vi "PXI_Host_LargeFXP_Write_OldMethod_Benchmark.vi"() -> ()   [LabVIEW 2018]
uses:
  <vilib>/Platform/TimedLoop/XDataNode/timing_clust.ctl
  <vilib>/Platform/TimedLoop/XDataNode/nitl_modes.ctl
  <vilib>/Platform/TimedLoop/XDataNode/wakeup.ctl
  <vilib>/NI/LVFPGA Adv Session Resources/OpenByNameSubVI.vi
  <vilib>/rvi/interface/common/dynamic/niFpgaEscapeDelimiterAndNull.vi
  <vilib>/Utility/error.llb/Error Cluster From Error Code.vi
  <vilib>/rvi/errors/niLvFpgaAdjustHostInterfaceError.vi
  <vilib>/FPGAPlugInAG/Dynamic/niLvFpga_Close_Dynamic.vi
  <vilib>/platform/TimedLoop/XDataNode/XDataNode.xnode
  <vilib>/NI/LVFPGA Adv Session Resources/OpenByName.xnode
  <vilib>/rvi/interface/nirviReadWriteControl/nirviReadWriteControl.xnode
  <vilib>/rvi/interface/nirviCloseFPGA/nirviCloseFPGA.xnode
  NiFpgaLv.dll
  <vilib>/rvi/interface/Simulation/niFpgaSimulationCallBeginRW.vi
  <vilib>/NI/LVFPGA Adv Session Resources/LVFPGAAdvSessionResources.lvlib
  cRIO RT/FPGA Bitfile Register Operations/Scalar IO Operations/FPGA Register IO.lvlib
  <vilib>/Platform/TimedLoop/XDataNode/XDNodeRunTimeDep.lvlib
panel:
  out "Maximum(s)":dbl
  out "Standard deviation":dbl
  out "Waveform Graph":dbl[](graph)
  out "error out":errorcluster
  out "Execution time (s)":dbl
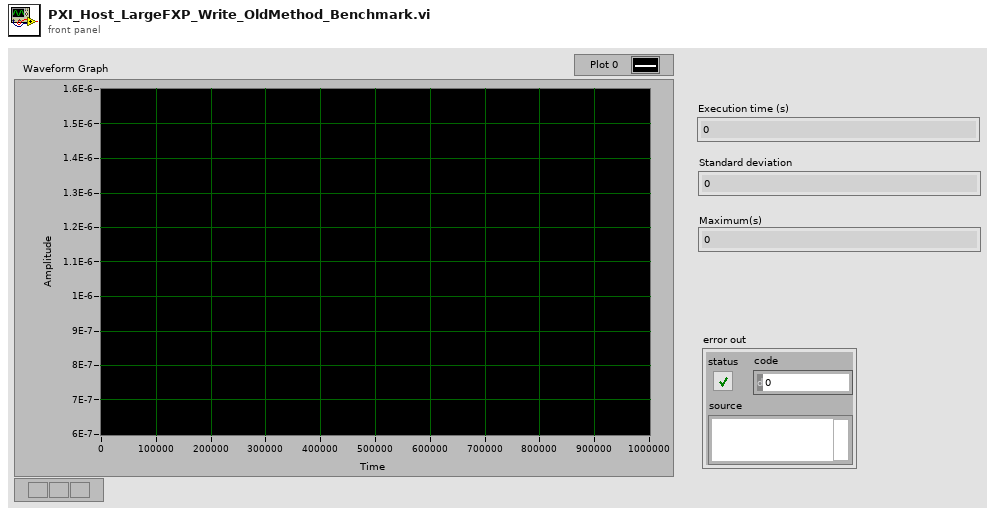
[diagram p1: front panel]
types:
  T1 = typedef "XDNodeRunTimeDep.lvlib/timing_clust.ctl" = cluster{"Expected End [f-1]":u64, "Actual End [f-1]":u64, "Finished Late? [f-1]":bool, "Expected End [i-1]":u64, "Actual End [i-1]":u64, "Finished Late? [i-1]":bool, "Expected Start [i]":u64, "Actual Start [i]":u64, "Expected Start [f]":u64, "Actual Start [f]":u64, "Source Name":string, "Structure Name":string, "Period":i64, "Deadline":i64, "Offset":i64, "Start":i64, "Priority":i32, "Timeout":i32, "Mode":T2, "Wakeup Reason":T3, "Error":errorcluster, "Source Type":string, "Secondary Source Type":string, "Global End Time":u64, "Global Start Time":u64, "Frame Duration":u64, "Iteration Duration":u64, "Assigned CPU":i32, "I/O Scan Engine Mode":u32}
  T2 = typedef "XDNodeRunTimeDep.lvlib/nitl_modes.ctl" = enum32{"No Change", "Process missed periods, maintain original phase", "Discard missed periods, maintain original phase", "Process missed periods, ignore original phase", "Discard missed periods, ignore original phase"}
  T3 = typedef "XDNodeRunTimeDep.lvlib/wakeup.ctl" = enum32{"Normal", "Aborted", "Asynchronous wakeup", "Timing source error", "Timed loop error", "Timeout"}
  T4 = cluster{"Name":string, "Depth":u32, "Write? (Deprecated:Use Implementation)":bool, "Physical Channel":u32, "Base Address":u32, "Data Width":u32, "Data Type":enum32{"Boolean", "I8", "I16", "I32", "I64", "U8", "U16", "U32", "U64", "FXP", "CustomControl", "SGL"}, "FXP Properties":variant, "Write Window Address":u32, "Implementation":enum16{"niFpgaTargetToHost", "niFpgaHostToTarget", "niFpgaPeerToPeerWriter", "niFpgaPeerToPeerReader", "niCoreTargetToHost", "niCoreHostToTarget"}, "Control Set":u32}[]
  T5 = cluster{"Name":string, "type":variant, "indicator?":bool}[]
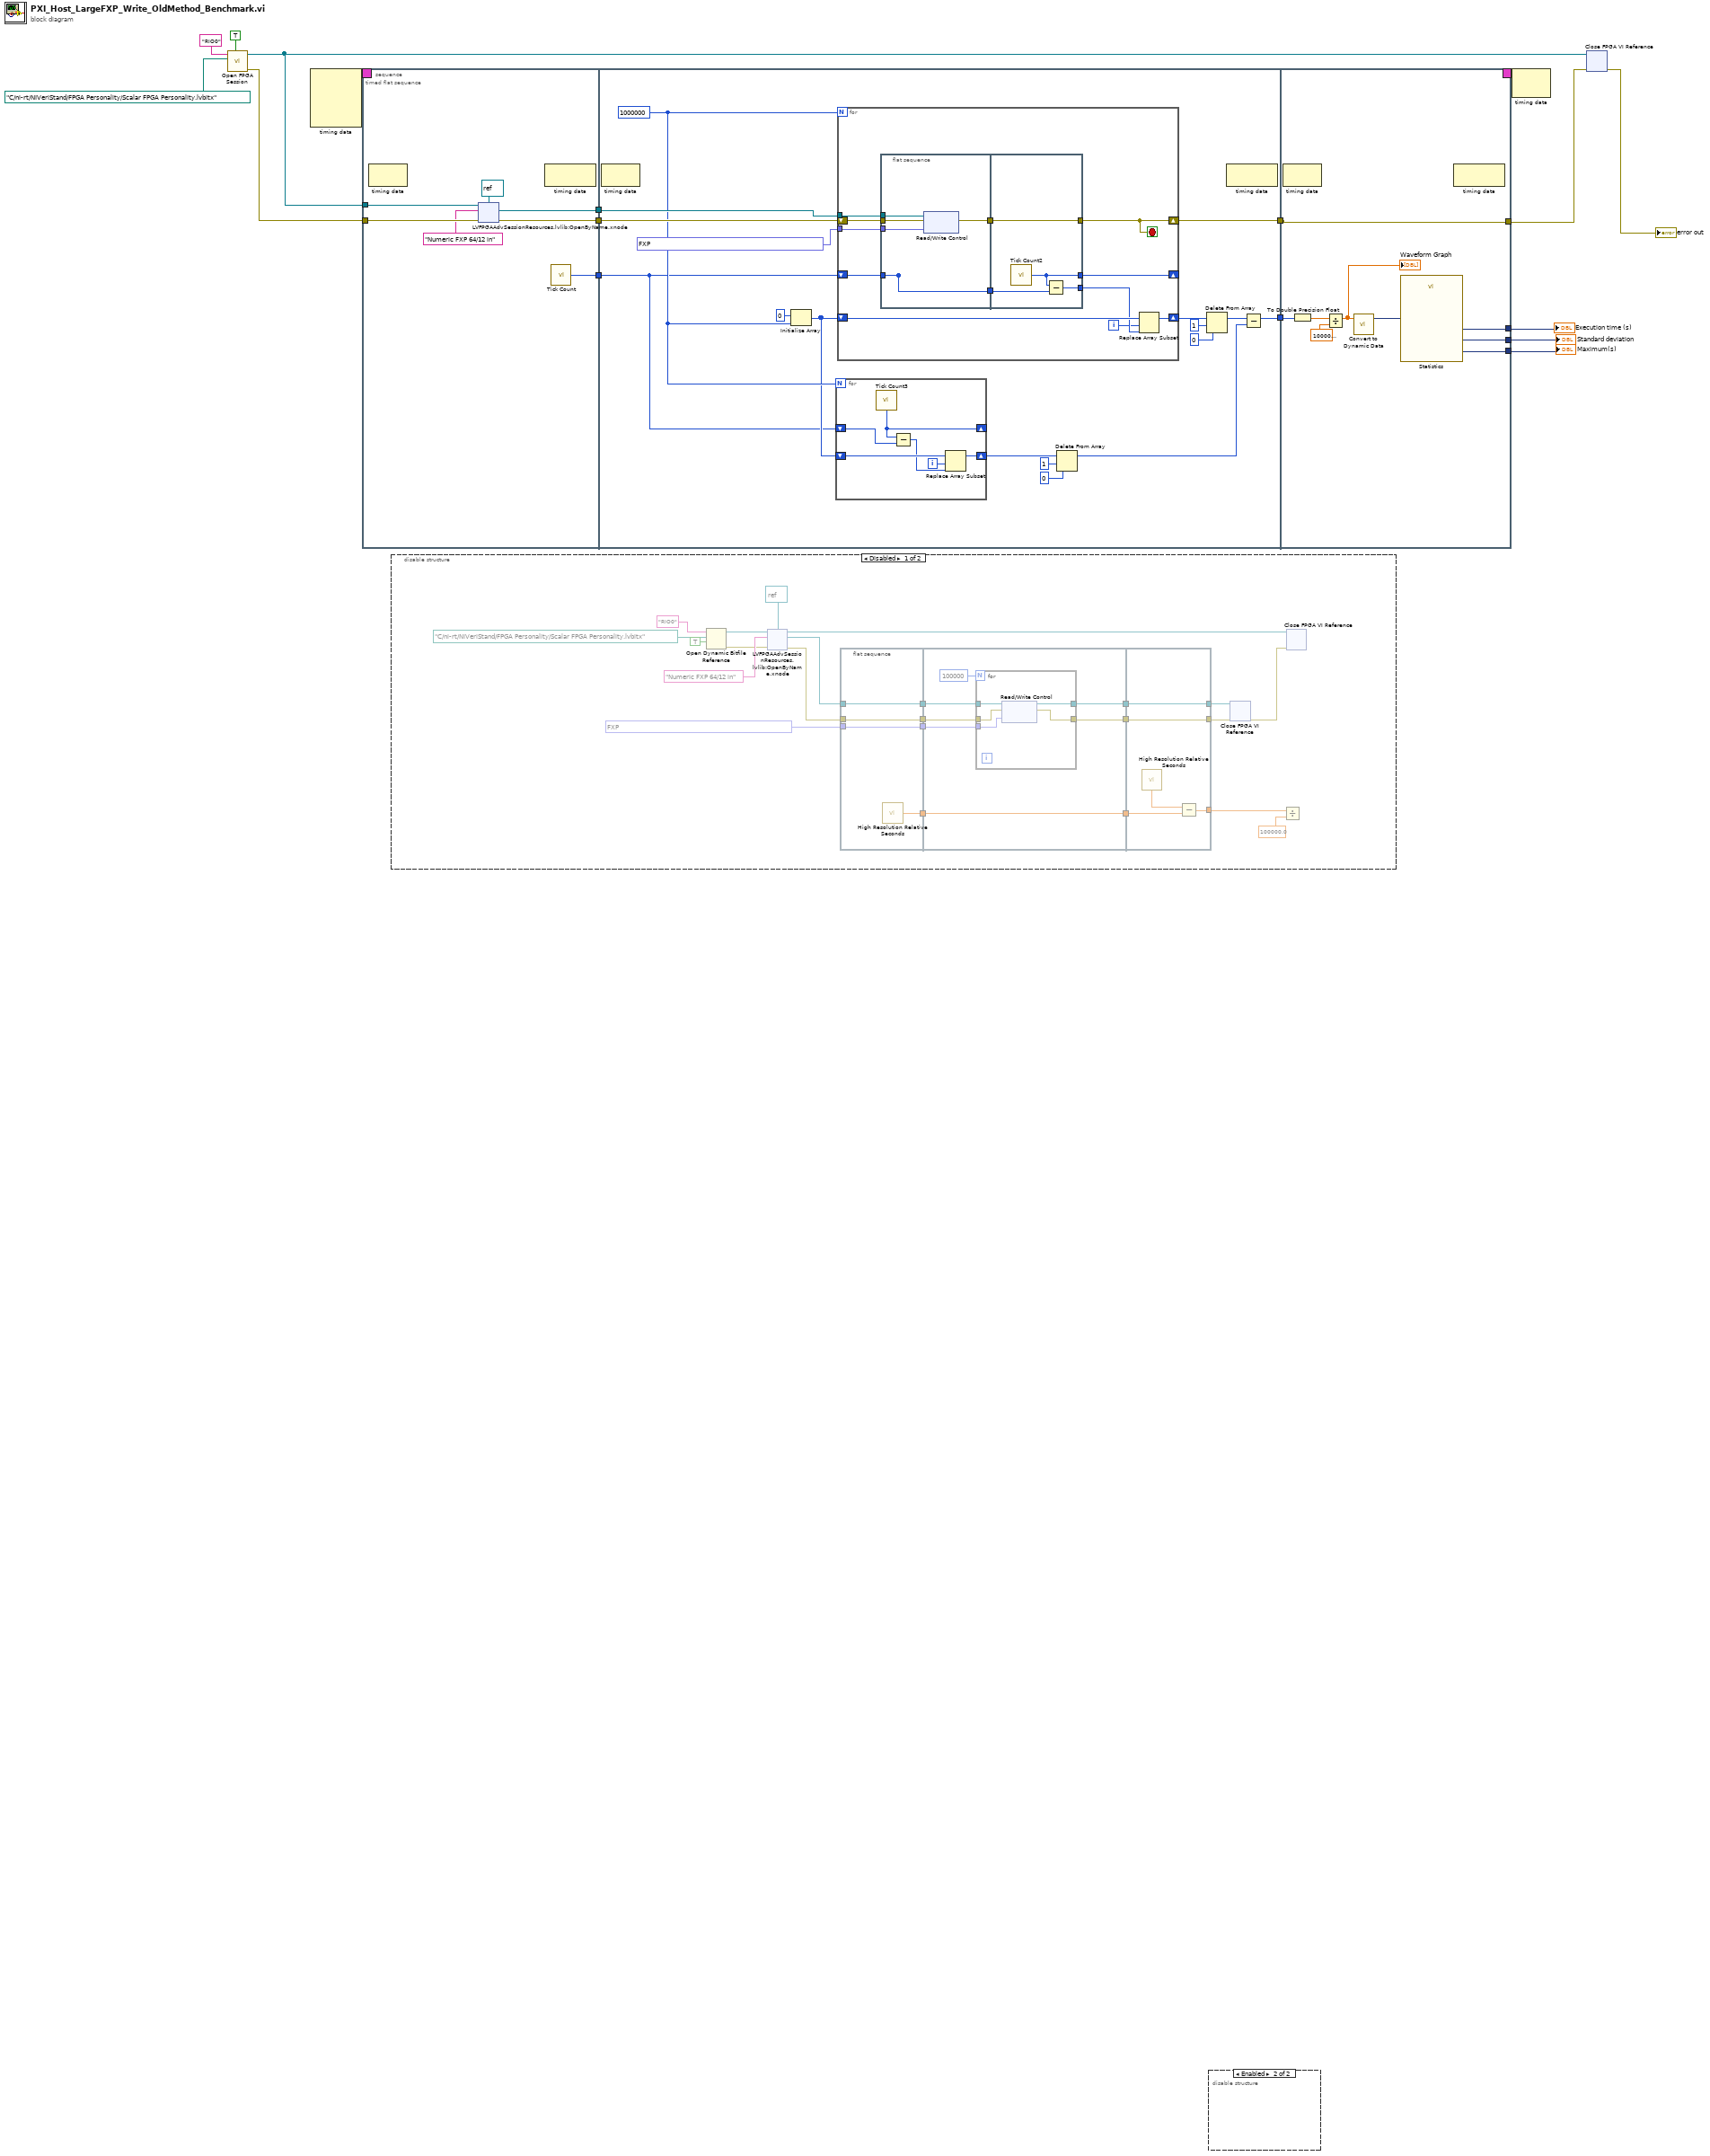
[diagram p0: block diagram]
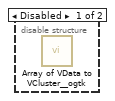
[diagram p3: hidden frame]
diagram:
  n1 = call "Open FPGA Session.vi"("run when loaded (T)"=TRUE, "bitfile path"=path "C:/ni-rt/NIVeriStand/FPGA Personality/Scalar FPGA Personality.lvbitx", "device address"="RIO0") -> ("error out"=w7:errorcluster, "bitfile reference out"=w1:refnum<k20>)  [unwired: 6 in, 1 out]
  n2 = node-c288() -> (w12:T1)  [unwired: 4 in]
  n3 = timed-sequence {
    timing: w12 -> [_]
    timing-out: [_] -> w11
    tunnel: w7 -> [w14]
    tunnel: [w20] -> w6
    tunnel: [w17] -> w4
    tunnel: [w16] -> w3
    tunnel: [w15] -> w2
    tunnel: w1 -> [w13]
    n4 = timed-flat-sequence {
      tunnel: [w27] -> w23
      tunnel: [w28] -> w22
      tunnel: [w30] -> w19
      tunnel: w14 -> [w26]
      tunnel: w13 -> [w29]
      tunnel: w23 -> [w62]
      tunnel: [w61] -> w21
      tunnel: w22 -> [w60]
      tunnel: w19 -> [w50]
      tunnel: [w47] -> w18
      tunnel: w21 -> [w100]
      tunnel: [w100] -> w20
      tunnel: w18 -> [w99]
      tunnel: [w97] -> w17
      tunnel: [w94] -> w16
      tunnel: [w93] -> w15
      frame #0 {
        n5 = node-c288() -> ()  [unwired: 1 in, 1 out]
        n6 = xnode "LVFPGAAdvSessionResources.lvlib:OpenByName.xnode"("FPGA VI Reference in"=w29, "Resource name in"="Numeric FXP 64/12 in", "Single resource reference type in"=refnum<k20> refnum ("Type"), "Error in"=w26) -> ("Single resource reference out"=w28:refnum<k20>, "Error out"=w27:errorcluster)  [unwired: 1 out]
        n7 = node-c288() -> ()  [unwired: 1 in, 1 out]
        n8 = call "Tick Count"() -> ("Tick Count(Ticks)"=w30:u32)
      }
      frame #1 {
        w52 = 1000000
        n9 = node-c288() -> ()  [unwired: 1 in, 1 out]
        n10 = Initialize Array(u32 0, w52) -> (w51:u32[])
        n11 = for {
          N: w52 -> [_]
          shift-right: [w63] -> w53
          shift-left: w51 -> [w66]
          shift-right: [w68] -> _
          shift-left: w50 -> [w67]
          i -> [w64]
          n12 = call "Tick Count3"() -> ("Tick Count(Ticks)"=w68:u32)
          n13 = Subtract(x=w68, y=w67) -> (x-y=w65:u32)
          n14 = Replace Array Subset(array=w66, new element=w65, index=w64) -> (w63:u32[])
        }
        n15 = for {
          N: w52 -> [_]
          tunnel: w60 -> [w81]
          shift-right: [w79] -> _
          shift-left: w50 -> [w78]
          shift-right: [w74] -> w58
          shift-left: w51 -> [w76]
          shift-right: [w72] -> w61
          shift-left: w62 -> [w82]
          tunnel: fxp<+/-,64,12> dbl? 5.371284094389756e+69 ("Value") -> [w71]
          i -> [w73]
          stop <- w72 stop-if-true
          n16 = flat-sequence {
            tunnel: w82 -> [w86]
            tunnel: w81 -> [w84]
            tunnel: [w85] -> w80
            tunnel: [w87] -> _
            tunnel: w78 -> [w87]
            tunnel: [w87] -> w77
            tunnel: w71 -> [w83]
            tunnel: [w91] -> w72
            tunnel: w80 -> [w91]
            tunnel: [w90] -> w79
            tunnel: w77 -> [w89]
            tunnel: [w88] -> w75
            frame #0 {
              n17 = xnode "Read/Write Control"("FPGA VI Reference In"=w84, "error in"=w86, "Value"=w83) -> ("error out"=w85:errorcluster)  [unwired: 1 out]
            }
            frame #1 {
              n18 = call "Tick Count2"() -> ("Tick Count(Ticks)"=w90:u32)
              n19 = Subtract(x=w90, y=w89) -> (x-y=w88:u32)
            }
          }
          n20 = Replace Array Subset(array=w76, new element=w75, index=w73) -> (w74:u32[])
        }
        n21 = Delete From Array(array=w53, length=1, index=0) -> (array with subset deleted=w48:u32[])  [unwired: 1 out]
        n22 = Delete From Array(array=w58, length=1, index=0) -> (array with subset deleted=w49:u32[])  [unwired: 1 out]
        n23 = node-c288() -> ()  [unwired: 1 in, 1 out]
        n24 = Subtract(x=w49, y=w48) -> (x-y=w47:u32[])
      }
      frame #2 {
        n25 = node-c288() -> ()  [unwired: 1 in, 1 out]
        n26 = To Double Precision Float(number=w99) -> (double precision float=w96:dbl[])
        n27 = Divide(x=w96, y=1000000000.0) -> (x/y=w92:dbl[])
        "Waveform Graph" <- w92
        n28 = call "Convert to Dynamic Data"("Array"=w92) -> ("Dynamic Data Type"=w98:dynamicdata)  [unwired: 3 in]
        n29 = call "Statistics"("Signals"=w98) -> ("Standard Dev"=w94:dynamicdata, "Arithmetic Mean"=w97:dynamicdata, "Maximum"=w93:dynamicdata)  [unwired: 23 in, 1 out]
        n30 = node-c288() -> ()  [unwired: 1 in, 1 out]
      }
    }
  }
  "Execution time (s)" <- w4
  "Standard deviation" <- w3
  "Maximum(s)" <- w2
  n31 = disable-structure shown="Disabled" {
    frame Disabled {
      n32 = Open Dynamic Bitfile Reference(0:"RIO0" ("Device address"), 1:path "C:/ni-rt/NIVeriStand/FPGA Personality/Scalar FPGA Personality.lvbitx" ("Bitfile path"), 2:TRUE ("Run When Loaded")) -> (5:w112:refnum<k20>, 8:w110:errorcluster)  [unwired: 2 in]
      n33 = xnode "LVFPGAAdvSessionResources.lvlib:OpenByName.xnode"("FPGA VI Reference in"=w112, "Resource name in"="Numeric FXP 64/12 in", "Single resource reference type in"=refnum<k20> refnum ("Type"), "Error in"=w110) -> ("Single resource reference out"=w108:refnum<k20>, "Error out"=w109:errorcluster, "FPGA VI Reference out"=w104:refnum<k20>)
      n34 = flat-sequence {
        tunnel: [w129] -> w125
        tunnel: w108 -> [w128]
        tunnel: [w128] -> w124
        tunnel: [w127] -> w123
        tunnel: w109 -> [w127]
        tunnel: [w126] -> w122
        tunnel: fxp<+/-,64,12> dbl? 5.371284094389756e+69 ("Value") -> [w126]
        tunnel: [w135] -> w121
        tunnel: w125 -> [w135]
        tunnel: w124 -> [w134]
        tunnel: w123 -> [w133]
        tunnel: [w132] -> w120
        tunnel: [w131] -> w119
        tunnel: w122 -> [w130]
        tunnel: w121 -> [w145]
        tunnel: [w144] -> w118
        tunnel: w120 -> [w143]
        tunnel: [w143] -> w113
        tunnel: w119 -> [w142]
        tunnel: [w142] -> w106
        frame #0 {
          n35 = call <vilib>:"High Resolution Relative Seconds.vi"() -> ("relative seconds"=w129:dbl)
        }
        frame #1 {
          n36 = for {
            N: 100000 -> [_]
            tunnel: w134 -> [w141]
            tunnel: w133 -> [w140]
            tunnel: [w139] -> w132
            tunnel: [w138] -> w131
            tunnel: w130 -> [w137]
            n37 = xnode "Read/Write Control"("FPGA VI Reference In"=w141, "error in"=w140, "Value"=w137) -> ("FPGA VI Reference Out"=w138:refnum<k20>, "error out"=w139:errorcluster)
          }
        }
        frame #2 {
          n38 = call <vilib>:"High Resolution Relative Seconds.vi"() -> ("relative seconds"=w146:dbl)
          n39 = Subtract(x=w146, y=w145) -> (x-y=w144:dbl)
        }
      }
      n40 = xnode "Close FPGA VI Reference"("FPGA VI Reference In"=w106, "error in"=w113) -> ("error out"=w105:errorcluster)
      n41 = Divide(x=w118, y=100000.0) -> ()  [unwired: 1 out]
      n42 = xnode "Close FPGA VI Reference"("FPGA VI Reference In"=w104, "error in"=w105) -> ()  [unwired: 1 out]
    }
    frame Enabled {
    }
  }
  n43 = disable-structure shown="Enabled" {
    frame Disabled {
      n44 = call <userlib>:"Array of VData to VCluster__ogtk.vi"() -> ()  [unwired: 10 in, 2 out]
    }
    frame Enabled {
    }
  }
  n45 = node-c288(w11) -> ()  [unwired: 1 out]
  n46 = xnode "Close FPGA VI Reference"("FPGA VI Reference In"=w1, "error in"=w6) -> ("error out"=→"error out":errorcluster)
